vi "RLC 电路频率特征曲线2.vi"() -> ()   [LabVIEW 2021]
panel:
  out "Waveform Graph":dynamicdata(graph)
  out "相-频曲线 2":cluster{"Y":dbl[], "Y":dbl[]}[](graph)
  out "幅-频曲线 2":cluster{"Y":dbl[], "Y":dbl[]}[](graph)
  out "ω0":dbl
  in  "C/μF":dbl
  in  "L/mH":dbl
  in  "R/Ω":dbl
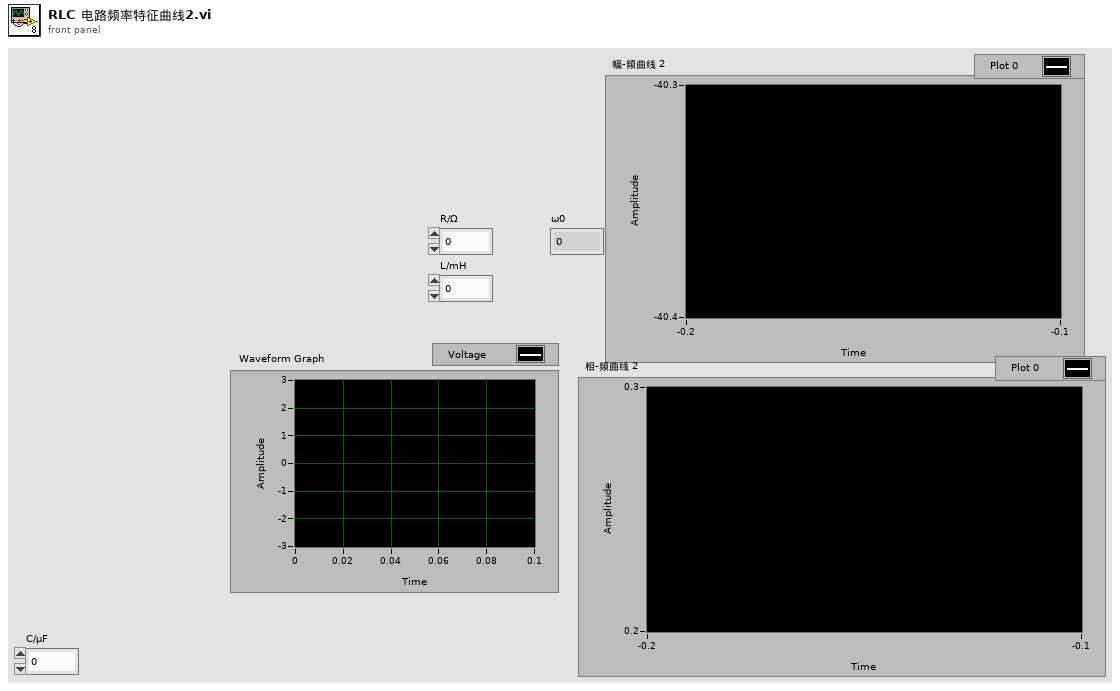
[diagram p1: front panel]
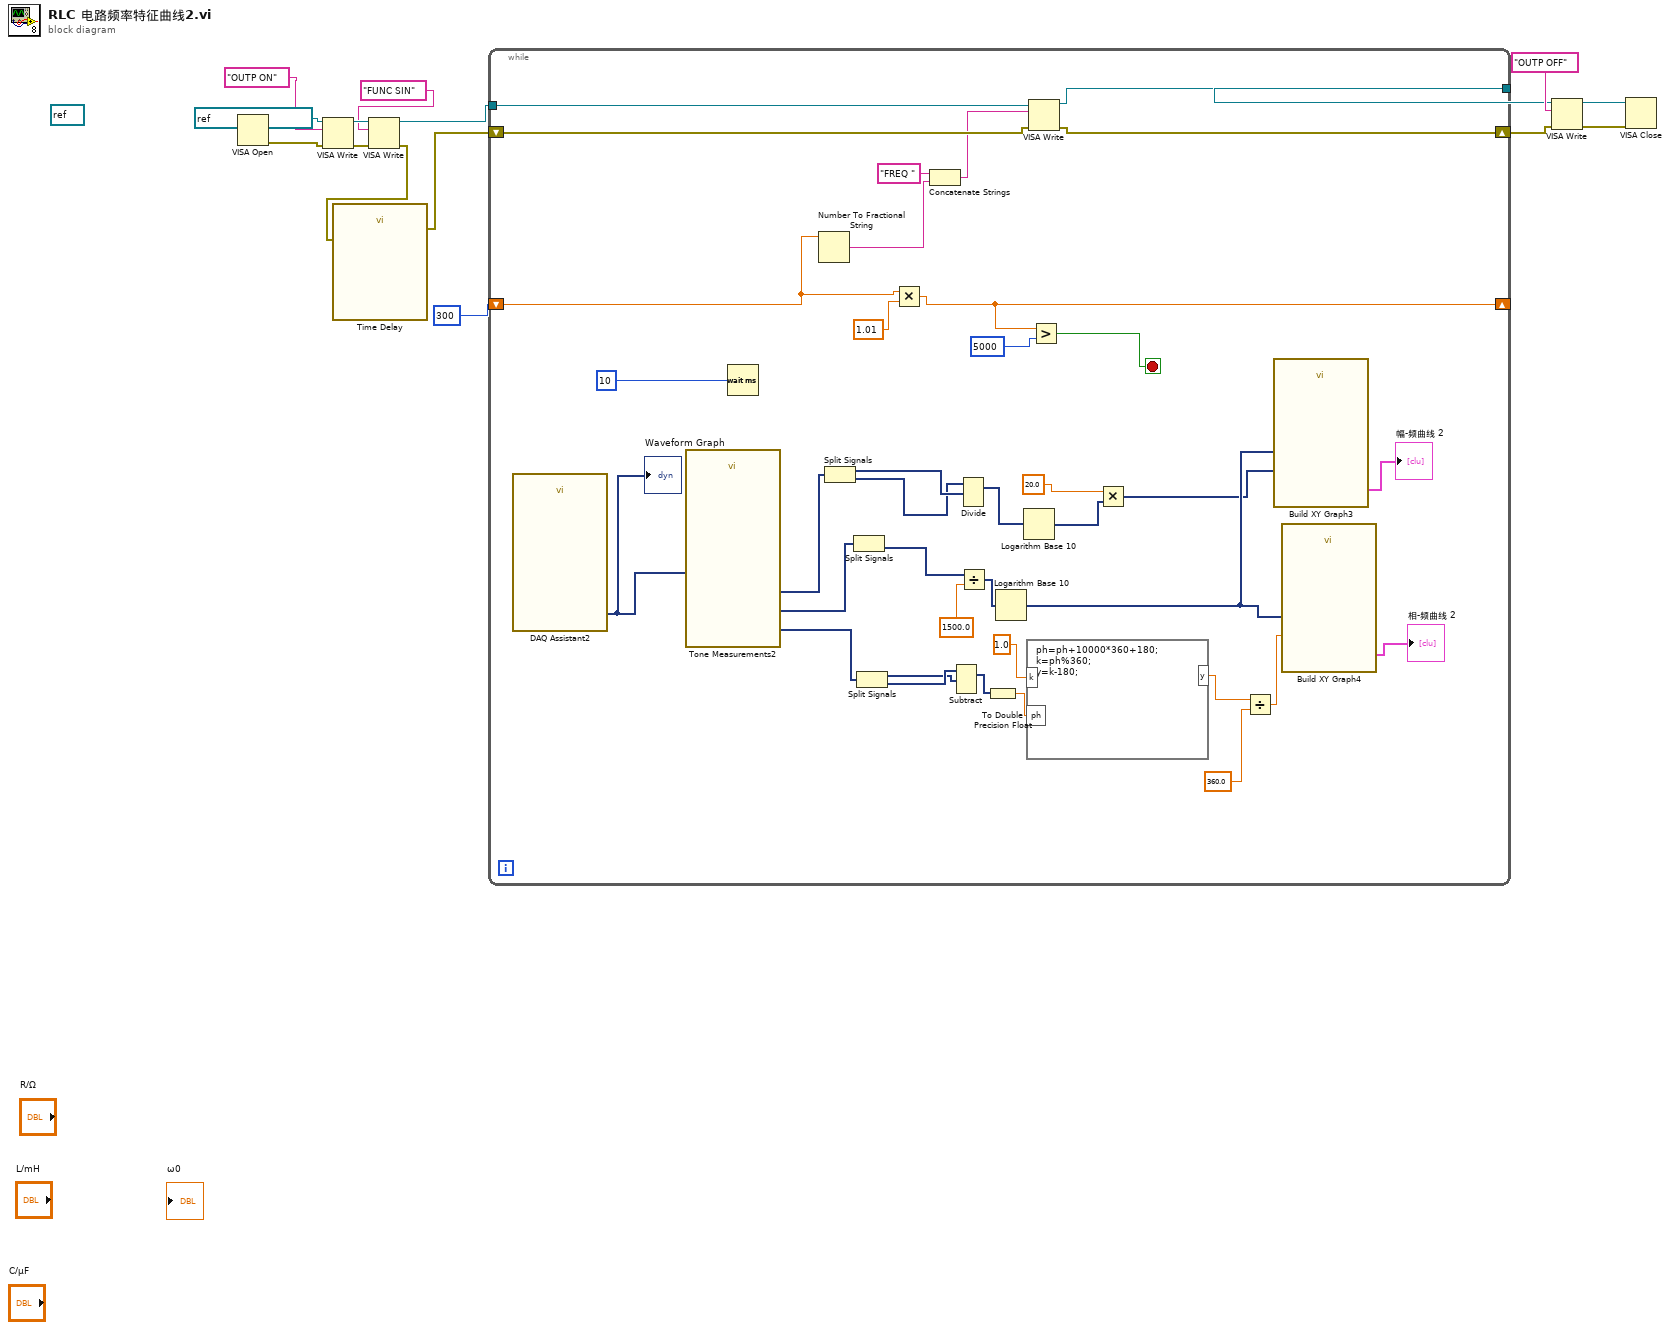
[diagram p0: block diagram]
diagram:
  (unwired) refnum<visa-resource-name> refnum ("VISA resource name")
  n1 = VISA Open(VISA resource name=refnum<visa-resource-name> "Rigol_DG1022U") -> (VISA resource name=w16:refnum<visa-resource-name>, error out=w15:errorcluster)  [unwired: 4 in]
  n2 = VISA Write(VISA resource name=w16, write buffer="OUTP ON", error in (no error)=w15) -> (VISA resource name out=w13:refnum<visa-resource-name>, error out=w11:errorcluster)  [unwired: 1 out]
  n3 = VISA Write(VISA resource name=w13, write buffer="FUNC SIN", error in (no error)=w11) -> (VISA resource name out=w7:refnum<visa-resource-name>, error out=w3:errorcluster)  [unwired: 1 out]
  n4 = call "Time Delay"("error in (no error)"=w3) -> ("error out"=w2:errorcluster)  [unwired: 10 in]
  n5 = while {
    tunnel: w7 -> [w53]
    tunnel: [w52] -> w6
    shift-right: [w50] -> w5
    shift-left: w2 -> [w51]
    shift-right: [w43] -> _
    shift-left: 300 -> [w44]
    stop <- w41 stop-if-true
    n6 = call "DAQ Assistant2"() -> ("data"=w25:dynamicdata)  [unwired: 17 in, 2 out]
    "Waveform Graph" <- w25
    n7 = call "Tone Measurements2"("Signals"=w25) -> ("Phase"=w22:dynamicdata, "Frequency"=w38:dynamicdata, "Amplitude"=w21:dynamicdata)  [unwired: 7 in, 1 out]
    n8 = Wait (ms)(milliseconds to wait=u32 10) -> ()  [unwired: 1 out]
    n9 = Number To Fractional String(number=w44) -> (F-format string=w47:string)  [unwired: 3 in]
    n10 = Split Signals(w21) -> (w34:dynamicdata, w33:dynamicdata)  [unwired: 2 in]
    n11 = Split Signals(w38) -> (w37:dynamicdata)  [unwired: 2 in, 1 out]
    n12 = Split Signals(w22) -> (w31:dynamicdata, w32:dynamicdata)  [unwired: 2 in]
    n13 = Multiply(x=w44, y=1.01) -> (x*y=w43:dbl)
    n14 = Concatenate Strings("FREQ " ("string"), w47) -> (w49:string)
    n15 = Subtract(1:w31, 2:w32) -> (0:w20:dynamicdata)  [unwired: 1 in, 1 out]
    n16 = Divide(1:w34, 2:w33) -> (0:w27:dynamicdata)  [unwired: 1 in, 1 out]
    n17 = Divide(x=w37, y=1500.0) -> (x/y=w36:dynamicdata)
    n18 = To Double Precision Float(number=w20) -> (double precision float=w24:dbl)
    n19 = Logarithm Base 10(1:w36) -> (0:w35:dynamicdata)
    n20 = Logarithm Base 10(1:w27) -> (0:w26:dynamicdata)
    n21 = formula code="ph=ph+10000*360+180;\nk=ph%360;\ny=k-180;"("ph"=w24, "k"=1.0) -> ("y"=w19:dbl)
    n22 = VISA Write(VISA resource name=w53, write buffer=w49, error in (no error)=w51) -> (VISA resource name out=w52:refnum<visa-resource-name>, error out=w50:errorcluster)  [unwired: 1 out]
    n23 = Greater?(x=w43, y=5000) -> (0:w41:bool)
    n24 = Multiply(x=20.0, y=w26) -> (x*y=w29:dynamicdata)
    n25 = Divide(x=w19, y=360.0) -> (x/y=w18:dbl)
    n26 = call "Build XY Graph3"("Y Input"=w29, "X Input"=w35) -> ("XY Graph"=→"幅-频曲线 2":cluster{"X":dbl[], "Y":dbl[]}[])  [unwired: 8 in, 1 out]
    n27 = call "Build XY Graph4"("Y Input"=w18, "X Input"=w35) -> ("XY Graph"=→"相-频曲线 2":cluster{"X":dbl[], "Y":dbl[]}[])  [unwired: 8 in, 1 out]
  }
  n28 = VISA Write(VISA resource name=w6, write buffer="OUTP OFF", error in (no error)=w5) -> (VISA resource name out=w9:refnum<visa-resource-name>, error out=w10:errorcluster)  [unwired: 1 out]
  n29 = VISA Close(VISA resource name=w9, error in (no error)=w10) -> ()  [unwired: 1 out]
